vi "transpozycja.vi"() -> ()   [LabVIEW 2024]
panel:
  out "out":dbl[][](array[numeric])
  out "transposed array":dbl[][](array[numeric])
  in  "in":dbl[][](array[numeric])
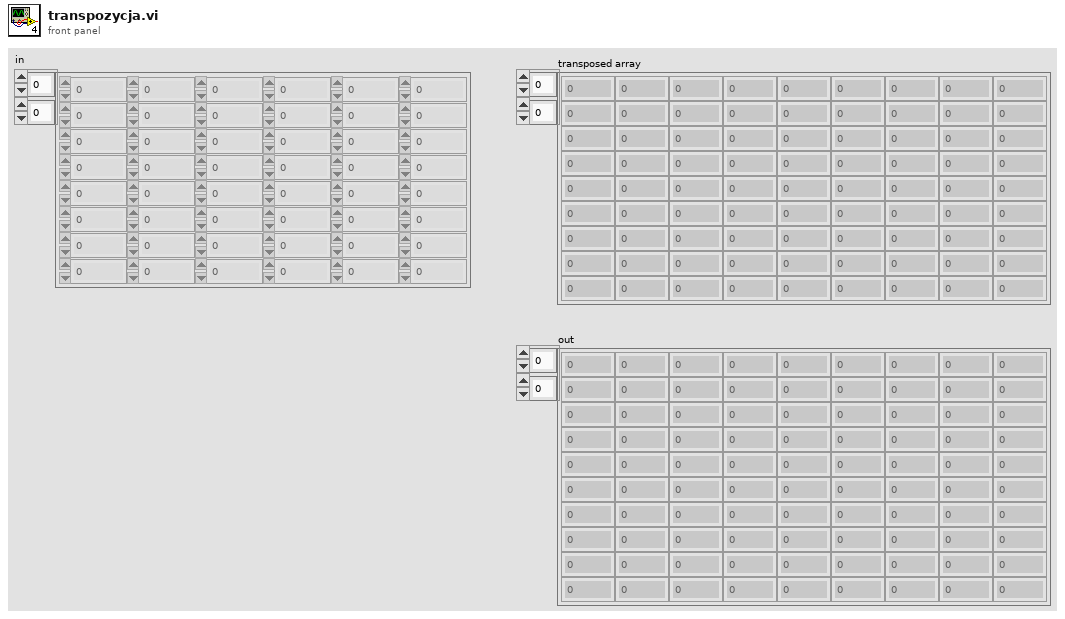
[diagram p1: front panel]
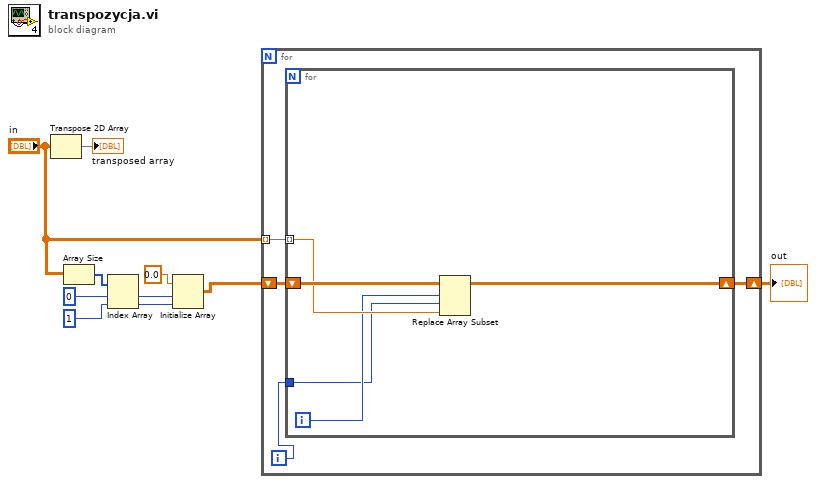
[diagram p0: block diagram]
diagram:
  n1 = Transpose 2D Array(2D array="in") -> (transposed array=→"transposed array":dbl[][])
  n2 = Array Size(array="in") -> (size(s)=w8:i32[])
  n3 = Index Array(array=w8, index #1=0 ("index"), index #2=1 ("index")) -> (element #1=w5:i32, element #2=w4:i32)
  n4 = Initialize Array(0.0 ("element"), w5, w4) -> (w3:dbl[][])
  n5 = for {
    tunnel: "in" -> [w14] mode=indexing
    shift-right: [w12] -> w1
    shift-left: w3 -> [w13]
    i -> [w11]
    n6 = for {
      tunnel: w14 -> [w17] mode=indexing
      shift-right: [w18] -> w12
      shift-left: w13 -> [w19]
      tunnel: w11 -> [w15]
      i -> [w16]
      n7 = Replace Array Subset(array=w19, new element=w17, index (row)=w16, index (col)=w15) -> (w18:dbl[][])
    }
  }
  "out" <- w1
